vi "rheodynevalve.vi"() -> ()   [LabVIEW 2019]
uses:
  Valve_class/Valve.lvclass
panel:
  in  "Exit":bool
  in  "Pos 2":bool
  in  "Pos1":bool
  in  "VISA resource name":refnum<visa-resource-name>
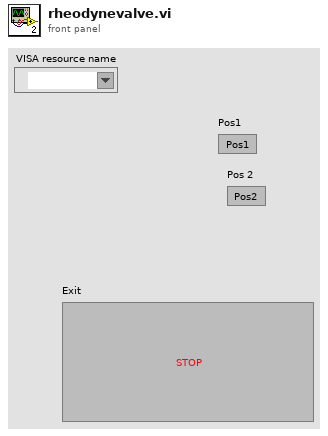
[diagram p1: front panel]
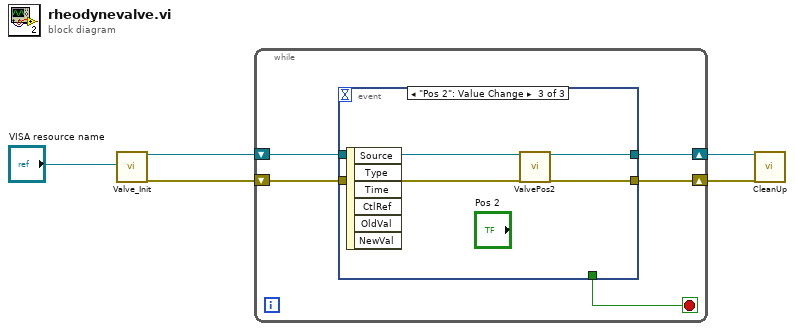
[diagram p0: block diagram]
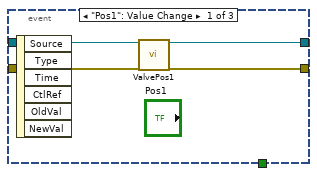
[diagram p2: hidden frame]
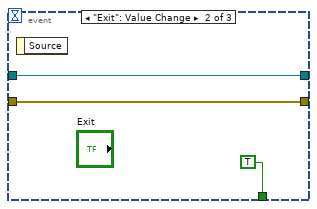
[diagram p3: hidden frame]
diagram:
  n1 = call "Valve_Init.vi"("VISA resource name"="VISA resource name") -> ("object out"=w4:refnum<class "Valve.lvclass">, "error out"=w3:errorcluster)  [unwired: 17 in]
  n2 = while {
    shift-right: [w7] -> w1
    shift-left: w4 -> [w10]
    shift-right: [w8] -> w2
    shift-left: w3 -> [w9]
    stop <- w6 stop-if-true
    n3 = event shown="[2] \"Pos 2\": Value Change" {
      selector: _ -> [_ _ _]
      dyn-events: _ -> [_ _ _]
      timeout: _ -> [_ _ _]
      tunnel: w10 -> [w14 w17 w21]
      tunnel: w9 -> [w13 w16 w20]
      tunnel: [w12 w16 w19] -> w8
      tunnel: [w11 w17 w18] -> w7
      tunnel: [_ TRUE _] -> w6
      event "Pos1": Value Change {
        n4 = event-data() -> ()  [unwired: 1 in, 6 out]
        n5 = call-dynamic "ValvePos1.vi"("object in"=w14, "error in (no error)"=w13) -> ("object out"=w11:refnum<class "Valve.lvclass">, "error out"=w12:errorcluster)  [unwired: 16 in]
      }
      event "Exit": Value Change {
        n6 = event-data() -> ()  [unwired: 1 in, 1 out]
      }
      event "Pos 2": Value Change {
        n7 = event-data() -> ()  [unwired: 1 in, 6 out]
        n8 = call-dynamic "ValvePos2.vi"("object in"=w21, "error in (no error)"=w20) -> ("object out"=w18:refnum<class "Valve.lvclass">, "error out"=w19:errorcluster)  [unwired: 16 in]
      }
    }
  }
  n9 = call-dynamic "CleanUp.vi"("object in"=w1, "error in (no error)"=w2) -> ()  [unwired: 16 in, 2 out]
